vi "Column I64.vi"(8 "error in (no error)":errorcluster, 11 "SQL Statement in":refnum<class "SQL Statement.lvclass">) -> (0 "error out":errorcluster, 2 "Int64":i64, 3 "SQL Statement out":refnum<class "SQL Statement.lvclass">)   [LabVIEW 2013, in "SQLiteSupport.lvlib" / "SQL Statement.lvclass"]
doc: "Returns the value in the next column as an I64 integer."
uses:
  SQL Statement.lvclass
  SQL Statement.lvclass/SQL Statement.ctl
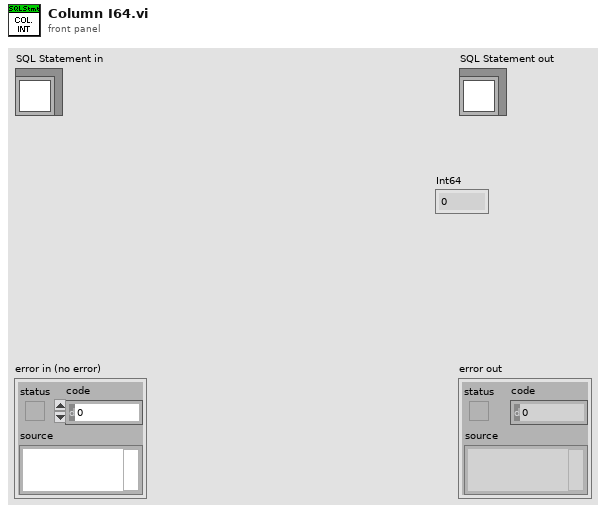
[diagram p1: front panel]
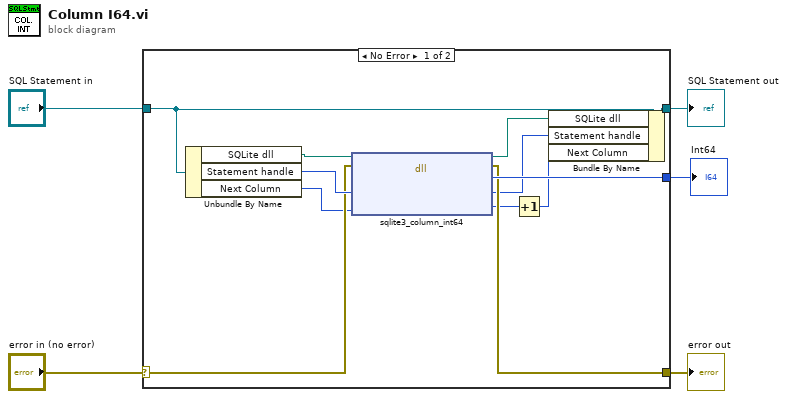
[diagram p0: block diagram]
diagram:
  n1 = case shown="No Error" "error in (no error)" {
    selector: "error in (no error)" -> [w15 w19]
    tunnel: [w12 w19] -> w4
    tunnel: [w10 w18] -> w2
    tunnel: "SQL Statement in" -> [w11 w18]
    tunnel: [w14 _] -> w1
    frame No Error {
      n2 = Unbundle By Name(w11) -> ("SQLite dll"=w17:path, "Statement handle"=w16:u64, "Next Column"=w13:i32)
      n3 = dll-call lib="C:/LabVIEW_JDP/Support/SQLite/sqlite3.dll" fn="sqlite3_column_int64"(path in=w17, error in=w15, "Statement"=w16, "Column"=w13) -> (path out=w6:path, error out=w12:errorcluster, "Int64"=w14:i64, "Statement"=w7:u64, "Column"=w9:i32)  [unwired: 1 in]
      n4 = Increment(x=w9) -> (x+1=w8:i32)
      n5 = Bundle By Name(cluster=w11, "SQLite dll"=w6, "Statement handle"=w7, "Next Column"=w8) -> (w10:refnum<class "SQL Statement.lvclass">)
    }
    frame Error {
    }
  }
  "error out" <- w4
  "SQL Statement out" <- w2
  "Int64" <- w1
